vi "ukol4.vi"() -> ()   [LabVIEW 2023]
uses:
  <vilib>/addons/Digital Filter Design/Process.llb/DFD Filtering (Wfm).vi
  <vilib>/measure/maspectr.llb/FFT Spectrum (Mag-Phase) for 1 Chan.vi
  <vilib>/measure/NI_MABase.lvlib
  <vilib>/addons/Digital Filter Design/NI_DigFilterLicensed.lvlib
  <vilib>/measure/NI_MAPro.lvlib
  <vilib>/Analysis/NI_AALPro.lvlib
panel:
  out "Waveform Graph 6":cluster{"f0":dbl, "df":dbl, "magnitude":dbl[]}[](graph)
  out "Waveform Graph 5":cluster{"f0":dbl, "df":dbl, "phase":dbl[]}[](graph)
  out "Waveform Graph 4":cluster{"f0":dbl, "df":dbl, "magnitude":dbl[]}[](graph)
  out "Waveform Graph 3":cluster{"f0":dbl, "df":dbl, "magnitude":dbl[]}[](graph)
  out "Waveform Graph 2":waveform(dbl)[](graph)
  out "Waveform Graph":waveform(dbl)[](graph)
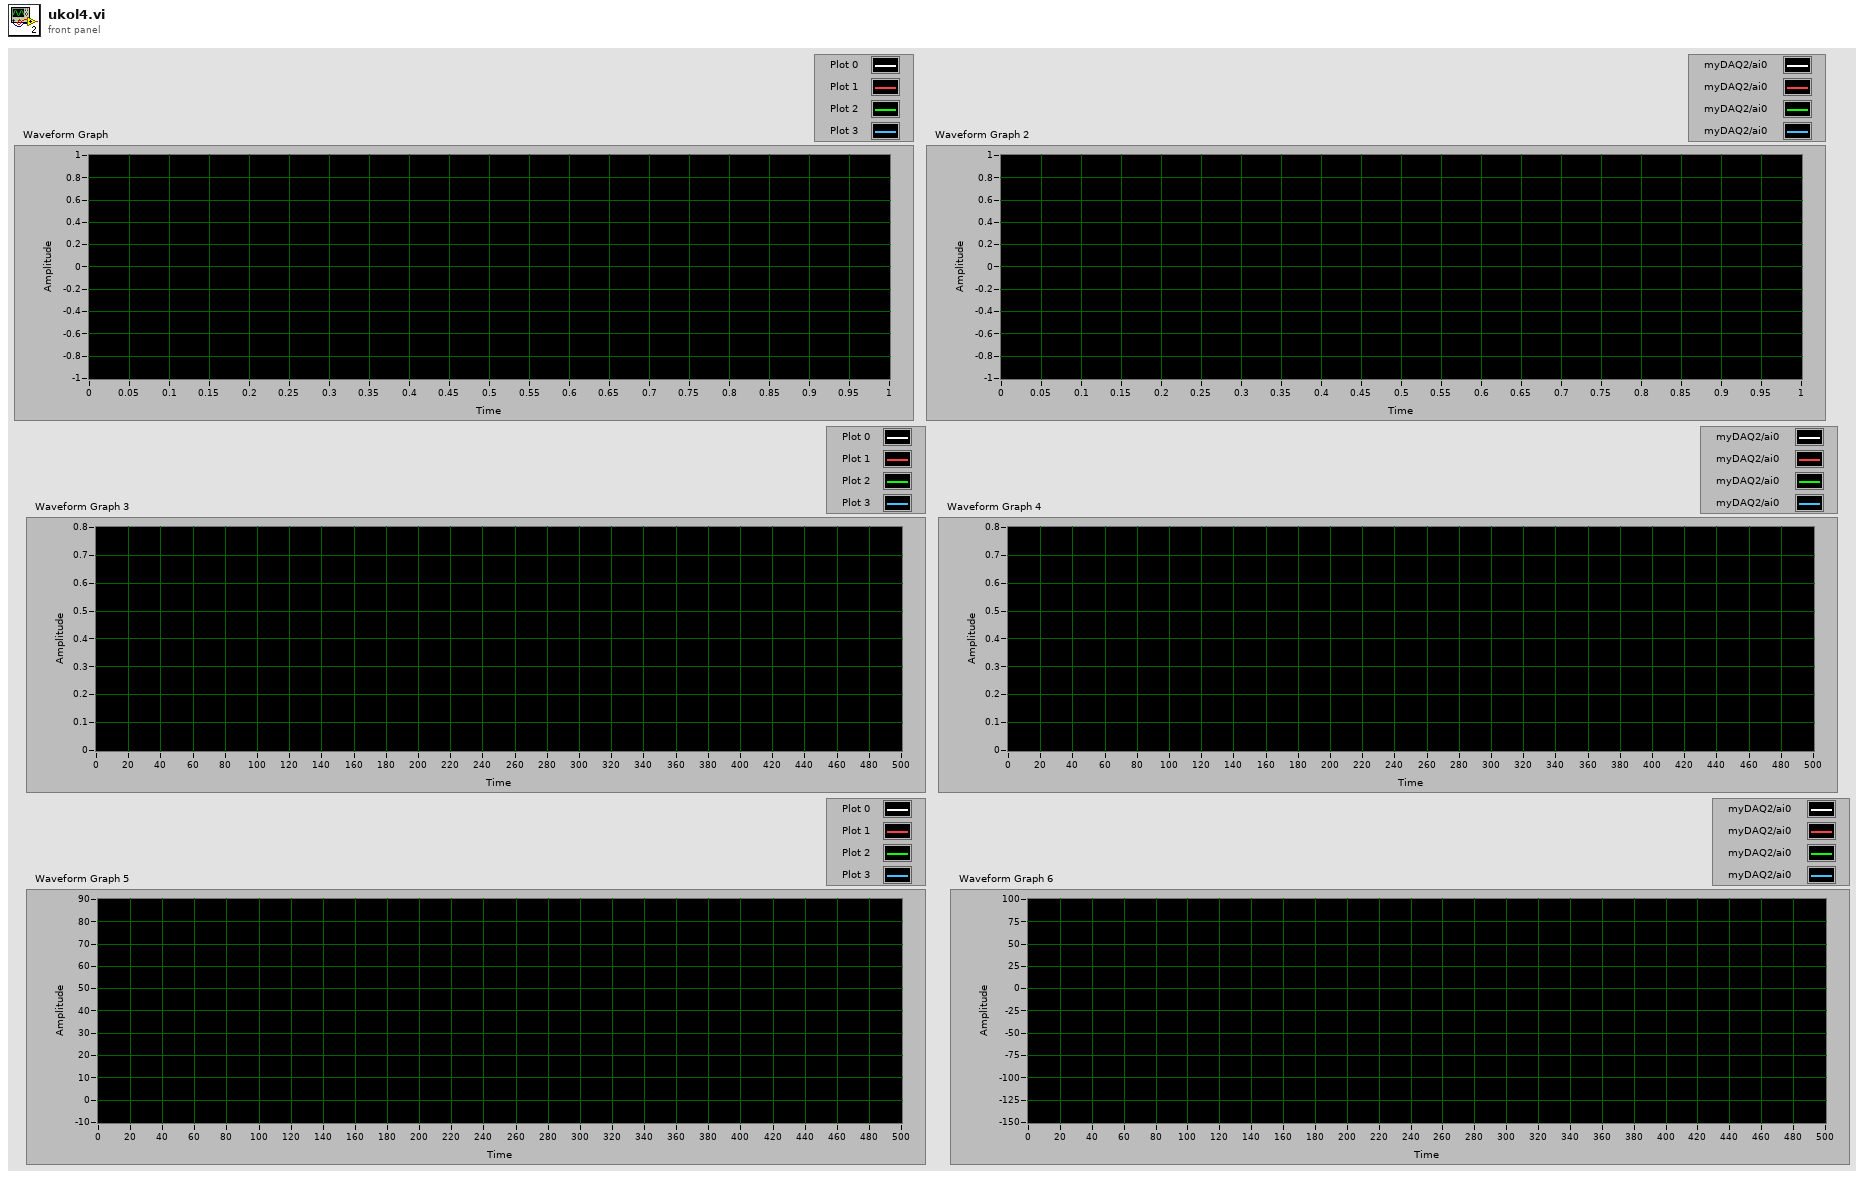
[diagram p1: front panel]
types:
  T1 = typedef "NI_DigFilterLicensed.lvlib/DFD Filter Obj.ctl" = cluster{"mSRate_Fs":dbl, "mSRate_Version":string, "mSRate_Comments":string, "mSRate_OrgCoef":T2, "mSRate_CurCoef":T2, "mSRate_Quantized?":bool, "mSRate_QCoef":T2, "mSRate_QSettings":T4[], "mSRate_Order":i32, "mSRate_Scaling":cluster{"mSRate_ScaleByPowerOf2?":bool, "mSRate_ScaleType":T6}}
  T2 = typedef "NI_DigFilterLicensed.lvlib/DFD Filter Coef.ctl" = cluster{"type":T3, "gain":dbl, "coef a (k)":dbl[], "coef b (v)":dbl[]}
  T3 = typedef "NI_DigFilterLicensed.lvlib/DFD Filter Structure Type Selector.ctl" = enum16{"Undefined", "FIR Direct Form", "FIR Direct Form Transposed", "FIR Symmetric", "FIR Antisymmetric", "IIR Direct Form I", "IIR Direct Form I Transposed", "IIR Direct Form II", "IIR Direct Form II Transposed", "IIR Cascaded Second Order Sections Form I", "IIR Cascaded Second Order Sections Form I Transposed", "IIR Cascaded Second Order Sections Form II", "IIR Cascaded Second Order Sections Form II Transposed", "Lattice Allpass (basic sections)", "Lattice Allpass (one multiplier sections)", "Lattice Allpass (normalized sections)", "Lattice AR (basic sections)", "Lattice AR (one multiplier sections)", "Lattice AR (normalized sections)", "Lattice MA (minimum phase)", "Lattice MA (maximum phase)", "Lattice ARMA (basic sections)", "Lattice ARMA (one multiplier sections)", "Lattice ARMA (normalized sections)"}
  T4 = typedef "NI_DigFilterLicensed.lvlib/dfd_Internal Quantization Settings.ctl" = cluster{"source":T5, "wl":i16, "iwl":i16, "overflow mode":enum16{"Saturation", "Wrap"}, "rounding mode":enum16{"Nearest", "Truncation"}, "signed?":bool}
  T5 = typedef "NI_DigFilterLicensed.lvlib/dfd_Internal Quantization Srcs.ctl" = u16
  T6 = typedef "NI_DigFilterLicensed.lvlib/DFD Coef Norm Type.ctl" = enum16{"No Norm", "Time Domain 1-Norm", "Time Domain 2-Norm", "Time Domain Inf-Norm"}
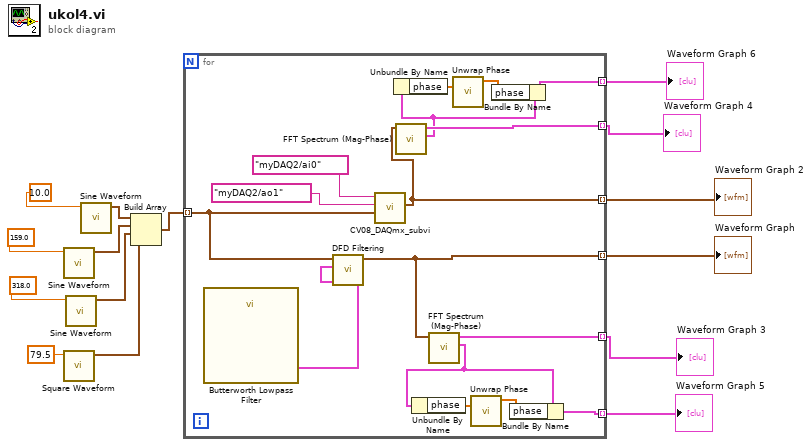
[diagram p0: block diagram]
diagram:
  n1 = call <vilib>:"Sine Waveform.vi"("frequency"=159.0) -> ("signal out"=w12:waveform(dbl))  [unwired: 9 in, 1 out]
  n2 = call <vilib>:"Square Waveform.vi"("frequency"=79.5) -> ("signal out"=w8:waveform(dbl))  [unwired: 9 in, 1 out]
  n3 = call <vilib>:"Sine Waveform.vi"("frequency"=318.0) -> ("signal out"=w10:waveform(dbl))  [unwired: 9 in, 1 out]
  n4 = call <vilib>:"Sine Waveform.vi"("frequency"=10.0) -> ("signal out"=w14:waveform(dbl))  [unwired: 9 in, 1 out]
  n5 = Build Array(w14, w12, w10, w8) -> (w9:waveform(dbl)[])
  n6 = for {
    tunnel: w9 -> [w29] mode=indexing
    tunnel: [w26] -> w6 mode=indexing
    tunnel: [w27] -> w5 mode=indexing
    tunnel: [w25] -> w4 mode=indexing
    tunnel: [w21] -> w3 mode=indexing
    tunnel: [w17] -> w2 mode=indexing
    tunnel: [w22] -> w1 mode=indexing
    n7 = call "Butterworth Lowpass Filter"() -> ("filter out"=w28:T1)  [unwired: 10 in, 1 out]
    n8 = call-poly <vilib>:"DFD Filtering.vi"("filter"=w28, "signal in"=w29) -> ("signal out"=w26:waveform(dbl))  [unwired: 8 in, 1 out]
    n9 = call "CV08_DAQmx_subvi.vi"("data in"=w29, "AO channel"=tag "myDAQ2/ao1", "AI channel"=tag "myDAQ2/ai0") -> ("data out"=w27:waveform(dbl))  [unwired: 7 in, 1 out]
    n10 = call-poly <vilib>:"FFT Spectrum (Mag-Phase).vi"("time signal"=w27) -> ("phase"=w20:cluster{"f0":dbl, "df":dbl, "phase":dbl[]}, "magnitude"=w21:cluster{"f0":dbl, "df":dbl, "magnitude":dbl[]})  [unwired: 6 in, 3 out]
    n11 = Unbundle By Name(w20) -> ("phase"=w24:dbl[])
    n12 = call-poly <vilib>:"FFT Spectrum (Mag-Phase).vi"("time signal"=w26) -> ("phase"=w16:cluster{"f0":dbl, "df":dbl, "phase":dbl[]}, "magnitude"=w25:cluster{"f0":dbl, "df":dbl, "magnitude":dbl[]})  [unwired: 6 in, 3 out]
    n13 = Unbundle By Name(w16) -> ("phase"=w19:dbl[])
    n14 = call <vilib>:"Unwrap Phase.vi"("Phase"=w24) -> ("Unwrapped Phase"=w23:dbl[])  [unwired: 9 in, 1 out]
    n15 = call <vilib>:"Unwrap Phase.vi"("Phase"=w19) -> ("Unwrapped Phase"=w18:dbl[])  [unwired: 9 in, 1 out]
    n16 = Bundle By Name(cluster=w20, "phase"=w23) -> (w22:cluster{"f0":dbl, "df":dbl, "phase":dbl[]})
    n17 = Bundle By Name(cluster=w16, "phase"=w18) -> (w17:cluster{"f0":dbl, "df":dbl, "phase":dbl[]})
  }
  "Waveform Graph" <- w6
  "Waveform Graph 2" <- w5
  "Waveform Graph 3" <- w4
  "Waveform Graph 4" <- w3
  "Waveform Graph 5" <- w2
  "Waveform Graph 6" <- w1
